vi "getState.vi"(8 "error in (no error)":errorcluster, 11 "Pump in":refnum<class "Pump.lvclass">) -> (0 "error out":errorcluster, 2 "state":bool, 3 "Pump out":refnum<class "Pump.lvclass">)   [LabVIEW 2020, in "Pump.lvclass"]
uses:
  Pump.lvclass
  Pump.lvclass/Pump.ctl
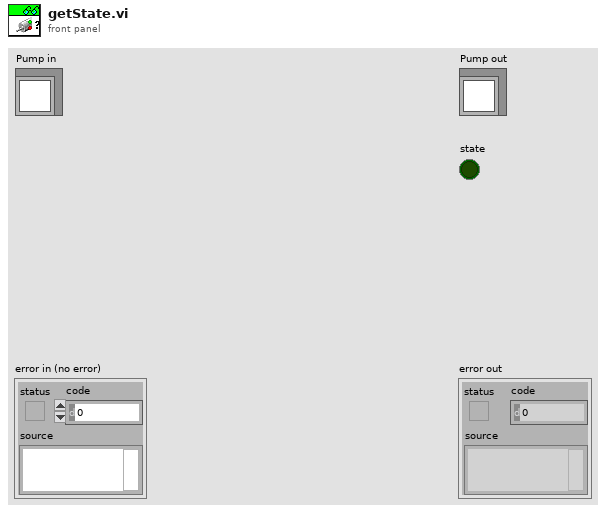
[diagram p1: front panel]
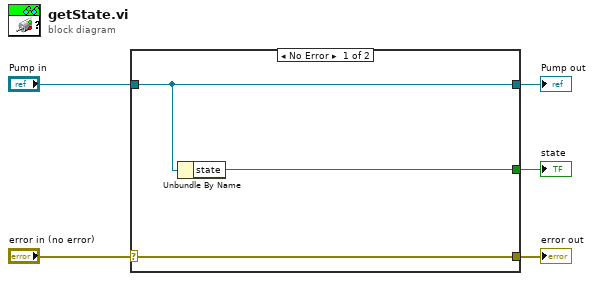
[diagram p0: block diagram]
diagram:
  n1 = case shown="No Error" "error in (no error)" {
    selector: "error in (no error)" -> [w8 w9]
    tunnel: [w8 w9] -> w4
    tunnel: [w7 w10] -> w2
    tunnel: "Pump in" -> [w7 w10]
    tunnel: [w6 _] -> w1
    frame No Error {
      n2 = Unbundle By Name(w7) -> ("state"=w6:bool)
    }
    frame Error {
    }
  }
  "error out" <- w4
  "Pump out" <- w2
  "state" <- w1
